vi "DIGITALDAQ.vi"(9 "error in":errorcluster, 10 "Canales":tag[](array[tag]), 11 "DAQ Board Name":tag) -> (2 "error out":errorcluster, 3 "task out":refnum<k21>)   [LabVIEW 2020, in "Acquisition.lvlib"]
uses:
  Acquisition.lvlib
  <vilib>/DAQmx/create/channels.llb/DAQmx Create Channel (DI-Digital Input).vi
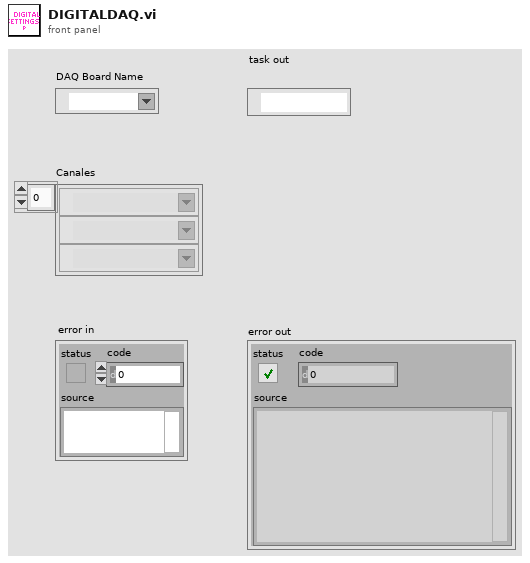
[diagram p1: front panel]
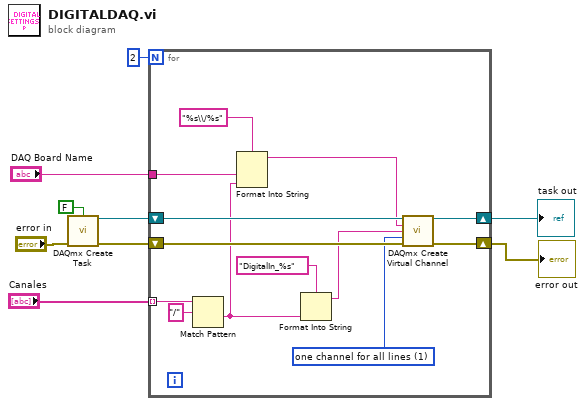
[diagram p0: block diagram]
diagram:
  n1 = call <vilib>:"DAQmx Create Task.vi"("auto cleanup"=FALSE, "error in"="error in") -> ("task out"=w7:refnum<k21>, "error out"=w8:errorcluster)  [unwired: 12 in]
  n2 = for {
    N: 2 -> [_]
    tunnel: "DAQ Board Name" -> [w20]
    tunnel: "Canales" -> [w19] mode=indexing
    shift-right: [w12] -> w3
    shift-left: w7 -> [w21]
    shift-right: [w11] -> w2
    shift-left: w8 -> [w22]
    w10 = 1 items=["one channel for each line", "one channel for all lines"] ("line grouping")
    n3 = Match Pattern(string=w19, regular expression="/") -> (after substring=w16:string)  [unwired: 1 in, 3 out]
    n4 = Format Into String(format string="%s\\/%s", w20, w16) -> (resulting string=w13:string)  [unwired: 2 in, 1 out]
    n5 = Format Into String(format string="DigitalIn_%s", w16) -> (resulting string=w14:string)  [unwired: 2 in, 1 out]
    n6 = call-poly <vilib>:"DAQmx Create Virtual Channel.vi"("task in"=w21, "lines"=w13, "name to assign"=w14, "line grouping"=w10, "error in"=w22) -> ("task out"=w12:refnum<k21>, "error out"=w11:errorcluster)  [unwired: 9 in]
  }
  "task out" <- w3
  "error out" <- w2
